vi "Write SystemConfigurationChange.vi"(8 "error in (no error)":errorcluster, 10 "SystemConfigurationChange":string, 11 "SystemConfiguration in":refnum<class "SystemConfiguration.lvclass">) -> (0 "error out":errorcluster, 3 "SystemConfiguration out":refnum<class "SystemConfiguration.lvclass">)   [LabVIEW 2019, in "SystemSetup.lvlib" / "SystemConfiguration.lvclass"]
uses:
  SystemConfiguration.lvclass
  SystemConfiguration.lvclass/SystemConfiguration.ctl
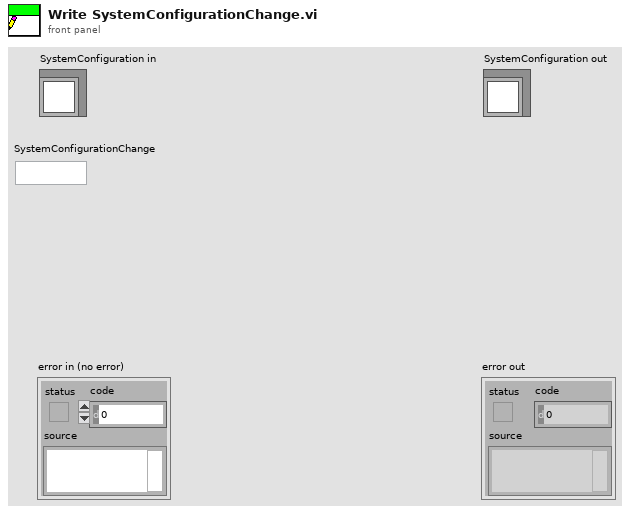
[diagram p1: front panel]
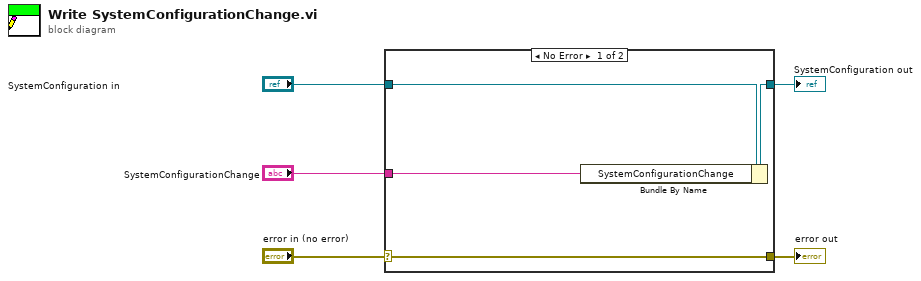
[diagram p0: block diagram]
diagram:
  n1 = case shown="No Error" "error in (no error)" {
    selector: "error in (no error)" -> [w9 w10]
    tunnel: [w9 w10] -> w4
    tunnel: [w7 w11] -> w2
    tunnel: "SystemConfiguration in" -> [w8 w11]
    tunnel: "SystemConfigurationChange" -> [w6 _]
    frame No Error {
      n2 = Bundle By Name(cluster=w8, "SystemConfigurationChange"=w6) -> (w7:refnum<class "SystemConfiguration.lvclass">)
    }
    frame Error {
    }
  }
  "error out" <- w4
  "SystemConfiguration out" <- w2
